vi "TargetUI.vi"() -> ()   [LabVIEW 2015, in "Target.lvclass"]
uses:
  Target.lvclass
  <vilib>/NI/Configuration Framework/Node/NodeRef.ctl
  <vilib>/NI/Configuration Framework/Node/NISE_CEF_Node.lvclass
  <vilib>/NI/AMC/Message Queue.ctl
  <vilib>/NI/AMC/Message.ctl
  <vilib>/NI/Tools/Keyed Array/KeyedArray.ctl
  <vilib>/NI/Configuration Framework/Node/UserEventRef.ctl
  <vilib>/NI/Configuration Framework/Controls/EventCluster.ctl
  Target.lvclass/Target.ctl
  Read Source.vi
  Write Source.vi
  <vilib>/NI/AMC/Create Single Message.vi
  <vilib>/NI/AMC/Update Message Routing Info.vi
  <vilib>/NI/AMC/Send Message.vi
  <vilib>/NI/AMC/AMC.lvlib
  Configuration Tool.lvlib
  <vilib>/NI/Tools/Keyed Array/Tools_KeyedArray.lvlib
  <vilib>/NI/Configuration Framework/NISE_CEF_TreeControl.lvlib
panel:
  in  "Real Time System Destination":string
  in  "Host Path to RT Driver VI":path
  in  "user event":T1
  in  "main queue":T2
  in  "node ref":T3
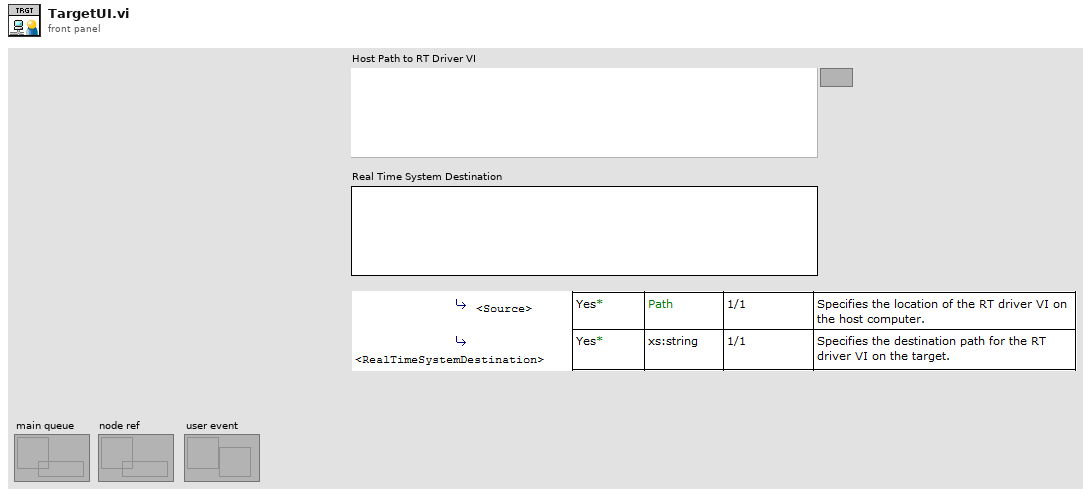
[diagram p1: front panel]
types:
  T1 = typedef "NISE_CEF_Node.lvclass/UserEventRef.ctl" = refnum<user-event>
  T2 = typedef "AMC.lvlib/Message Queue.ctl" = refnum<queue>
  T3 = typedef "NISE_CEF_Node.lvclass/NodeRef.ctl" = refnum<data-value>
  T4 = typedef "VeriStand Custom Device XML Parser.lvlib/Path Cluster.ctl" = cluster{"Path":path, "Path Type":enum16{"Absolute", "To Base", "To Common Doc Dir", "To Application Data Dir"}}
  T5 = typedef "VeriStand Custom Device XML Parser.lvlib/Supported Targets.ctl" = enum16{"All", "Pharlap", "VxWorks", "Windows", "Linux_32_ARM", "Linux_x64", "PharlapWindows", "PharlapVxWorks", "VxWorksWindows"}
  T6 = cluster{"Source":T4, "Real Time System Destination":string, "Supported Target":T5}
  T7 = enum16{"Absolute", "To Base", "To Common Doc Dir", "To Application Data Dir"}
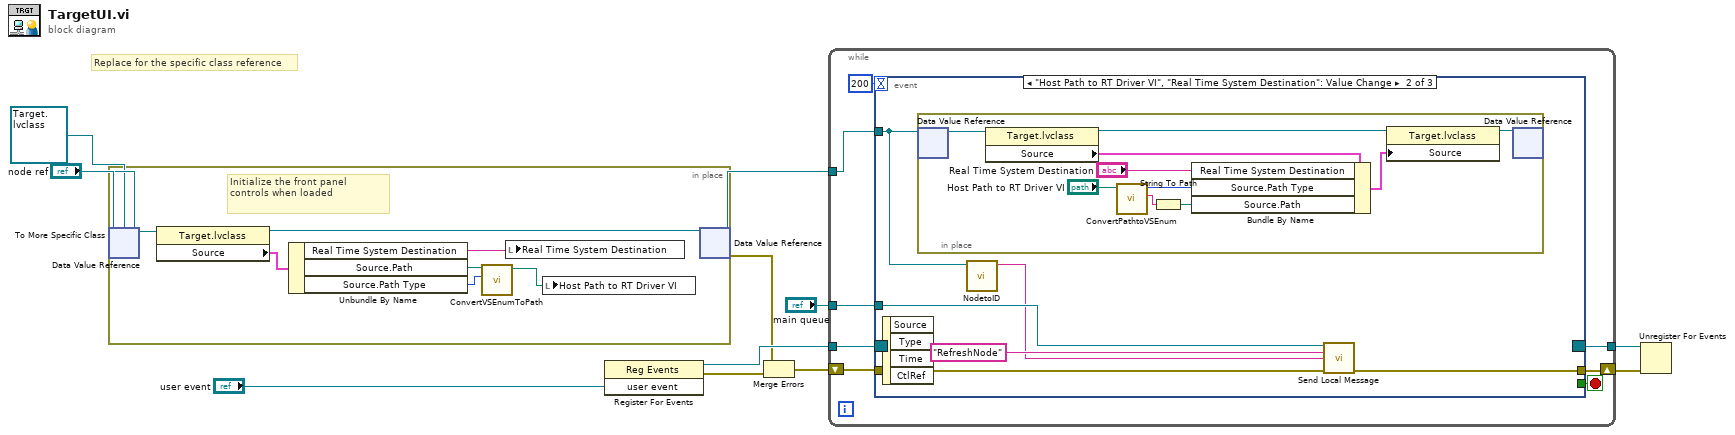
[diagram p0: block diagram]
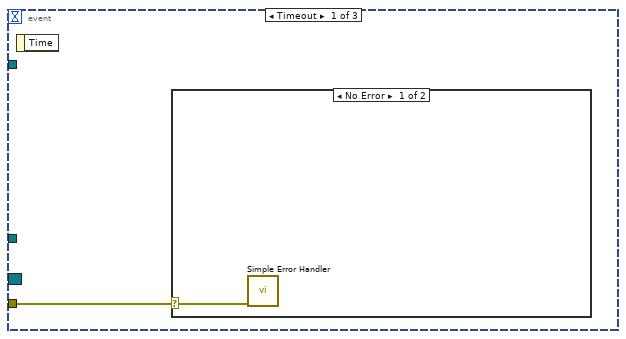
[diagram p2: hidden frame]
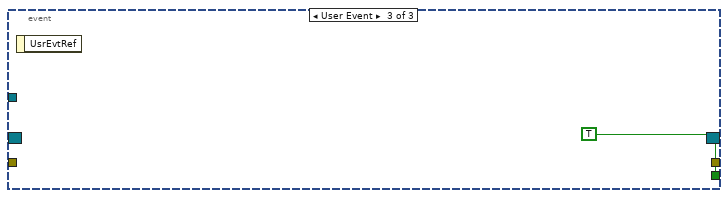
[diagram p4: hidden frame]
diagram:
  # "Replace for the specific class reference"
  n1 = To More Specific Class(target class=refnum<data-value> refnum ("data value reference"), reference="node ref") -> (specific class reference=w5:refnum<data-value>)  [unwired: 1 in, 1 out]
  n2 = in-place {
    # "Initialize the front panel controls when loaded"
    n3 = in-place-dvr #1(w5) -> (w19:refnum<class "Target.lvclass">)  [unwired: 1 out]
    n4 = property class="Target.lvclass"(reference=w19) -> (reference out=w18:refnum<class "Target.lvclass">, "Source"=w13:T6)  [unwired: 1 in, 1 out]
    n5 = Unbundle By Name(w13) -> ("Real Time System Destination"=w15:string, "Source.Path"=w17:path, "Source.Path Type"=w16:T7)
    n6 = call "ConvertVSEnumToPath.vi"("Source.Path Type"=w16, "Path In"=w17) -> ("appended path"=w14:path)  [unwired: 9 in]
    n7 = local write "Real Time System Destination"(w15) -> ()
    n8 = local write "Host Path to RT Driver VI"(w14) -> ()
    n9 = in-place-dvr #1(w18) -> (w12:refnum<data-value>, w2:errorcluster)
  }
  n10 = register-events("user event") -> (reference out=w9:refnum<event-registration>, error out=w3:errorcluster)  [unwired: 2 in]
  n11 = Merge Errors(w2, w3) -> (w1:errorcluster)
  n12 = while {
    tunnel: w12 -> [w27]
    tunnel: "main queue" -> [w26]
    tunnel: w9 -> [w24]
    tunnel: [w23] -> w8
    shift-right: [w21] -> w7
    shift-left: w1 -> [w20]
    stop <- w22 stop-if-true
    n13 = event shown="[1] \"Host Path to RT Driver VI\", \"Real Time System Destination\": Value Change" {
      selector: w24 -> [_ _ _]
      dyn-events: [_ _ _] -> w23
      timeout: 200 -> [_ _ _]
      tunnel: w27 -> [_ w33 _]
      tunnel: w26 -> [_ w34 _]
      tunnel: [_ _ TRUE] -> w22
      tunnel: [_ w31 _] -> w21
      tunnel: w20 -> [w28 w30 _]
      event Timeout {
        n14 = event-data() -> ()  [unwired: 1 in, 1 out]
        n15 = case shown="No Error" w28 {
          selector: w28 -> [w29 _]
          frame No Error {
            n16 = call <vilib>:"Simple Error Handler.vi"("error in (no error)"=w29) -> ()  [unwired: 4 in, 5 out]
          }
          frame Error {
          }
        }
      }
      event "Host Path to RT Driver VI", "Real Time System Destination": Value Change {
        n17 = event-data() -> ()  [unwired: 1 in, 4 out]
        n18 = in-place {
          n19 = in-place-dvr #2(w33) -> (w43:refnum<class "Target.lvclass">)  [unwired: 1 out]
          n20 = property class="Target.lvclass"(reference=w43) -> (reference out=w38:refnum<class "Target.lvclass">, "Source"=w42:T6)  [unwired: 1 in, 1 out]
          n21 = call "ConvertPathtoVSEnum.vi"("Path In"="Host Path to RT Driver VI") -> ("Remaining Path"=w36:string, "VS Enum Out"=w39:T7)  [unwired: 9 in]
          n22 = String To Path(string=w36) -> (path=w37:path)
          n23 = Bundle By Name(cluster=w42, "Real Time System Destination"="Real Time System Destination", "Source.Path Type"=w39, "Source.Path"=w37) -> (w41:T6)
          n24 = property class="Target.lvclass"(reference=w38, "Source"=w41) -> (reference out=w45:refnum<class "Target.lvclass">)  [unwired: 1 in, 1 out]
          n25 = in-place-dvr #2(w45) -> ()  [unwired: 2 out]
        }
        n26 = call <vilib>:"NodetoID.vi"("node ref"=w33) -> ("ID"=w32:string)  [unwired: 9 in, 1 out]
        n27 = call <vilib>:"Send Local Message.vi"("message queue in"=w34, "message name"="RefreshNode" ("Message Name"), "message value"=w32, "error in"=w30) -> ("error out"=w31:errorcluster)  [unwired: 9 in, 2 out]
      }
      event User Event {
        n28 = event-data() -> ()  [unwired: 1 in, 1 out]
      }
    }
  }
  n29 = Unregister For Events(event registration refnum=w8, error in=w7) -> ()  [unwired: 1 out]
